vi "Read send failure.vi"(8 "error in":errorcluster, 11 "MQTT client in":refnum<class "MQTT client.lvclass">) -> (0 "error out":errorcluster, 2 "send failure":refnum<event-registration>, 3 "MQTT client out":refnum<class "MQTT client.lvclass">)   [LabVIEW 2014, in "MQTT client.lvclass"]
uses:
  MQTT client.lvclass
  message acknowledgement.ctl
  MQTT client.lvclass/MQTT client.ctl
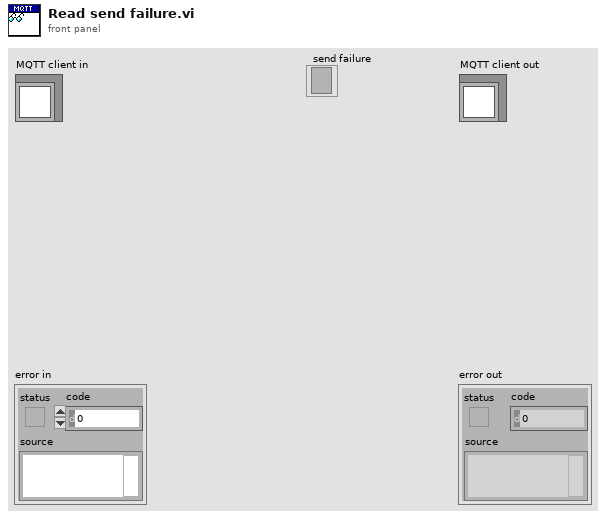
[diagram p1: front panel]
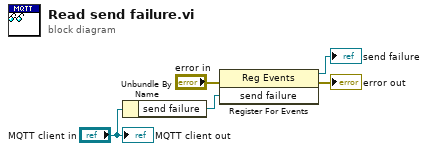
[diagram p0: block diagram]
diagram:
  n1 = Unbundle By Name("MQTT client in") -> ("send failure"=w2:refnum<user-event>)
  n2 = register-events(error in="error in", w2) -> (reference out=→"send failure":refnum<event-registration>, error out=→"error out":errorcluster)  [unwired: 1 in]
  "MQTT client out" <- "MQTT client in"
